vi "Start Animation.vi"(8 "Error In":errorcluster, 11 "Animation Config":T1) -> (0 "Error Out":errorcluster, 3 "Animation Config":T1)   [LabVIEW 2011, in "LMH-Toolbox.lvlib" / "LMH GUI Tools.lvlib"]
uses:
  LMH GUI Tools.lvlib
  Private/Animations/Type Defs/Animation Config.ctl
  <vilib>/picture/picture.llb/imagedata.ctl
  Private/Animations/FGVs/Type Defs/Animation FGV State.ctl
  LMH-Toolbox.lvlib
panel:
  in  "Error In 2":errorcluster
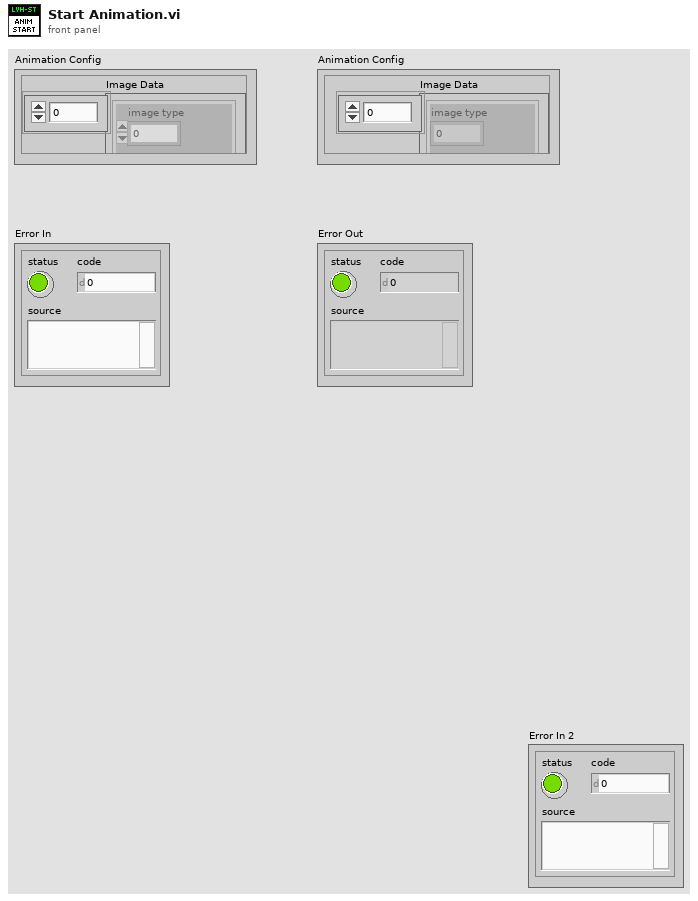
[diagram p1: front panel]
types:
  T1 = typedef "LMH-Toolbox.lvlib/LMH GUI Tools.lvlib/Animation Config.ctl" = cluster{"Image Data":T2[], "Animation Picture Indicator":refnum<vi>, "FPS":u32, "Position":cluster{"X":i16, "Y":i16}}
  T2 = typedef "imagedata.ctl" = cluster{"image type":i32, "image depth":i32, "image":u8[], "mask":u8[], "colors":u32[], "Rectangle":cluster{"left":i16, "top":i16, "right":i16, "bottom":i16}}
  T3 = enum32{"invalid app kind", "Development System", "Run Time System", "Student Edition", "Embedded LabVIEW", "Evaluation", "Custom"}
  T4 = typedef "LMH-Toolbox.lvlib/LMH GUI Tools.lvlib/Animation FGV State.ctl" = enum16{"Init", "Set", "Get"}
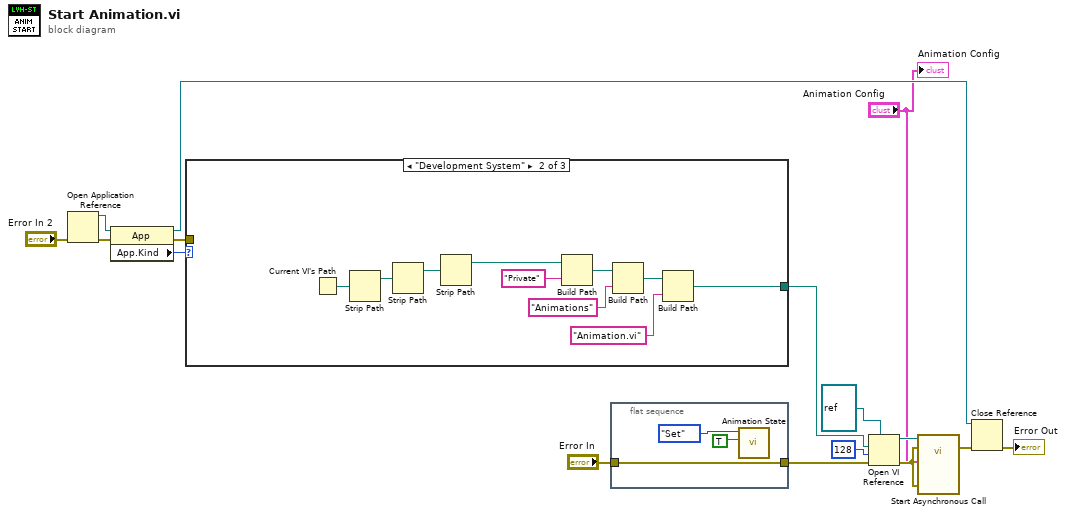
[diagram p0: block diagram]
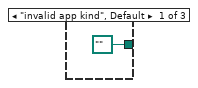
[diagram p2: hidden frame]
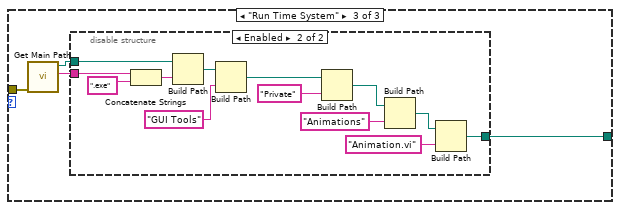
[diagram p3: hidden frame]
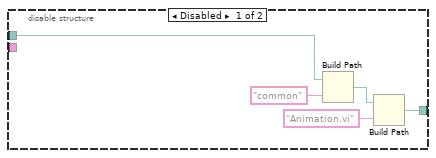
[diagram p4: hidden frame]
diagram:
  n1 = Open Application Reference(8:"Error In 2") -> (0:w11:errorcluster, 3:w10:refnum<vi>)  [unwired: 3 in]
  n2 = property class="App"(reference=w10, error in=w11) -> (reference out=w5:refnum<vi>, error out=w7:errorcluster, "App.Kind"=w9:T3)
  n3 = case shown="\"Development System\"" w9 {
    tunnel: [path "" ("appended path") w22 w29] -> w8
    tunnel: w7 -> [_ _ w30]
    frame "invalid app kind", Default {
    }
    frame "Development System" {
      n4 = Current VI's Path() -> (path=w27:path)
      n5 = Strip Path(path=w27) -> (stripped path=w24:path)  [unwired: 1 out]
      n6 = Strip Path(path=w24) -> (stripped path=w25:path)  [unwired: 1 out]
      n7 = Strip Path(path=w25) -> (stripped path=w19:path)  [unwired: 1 out]
      n8 = Build Path(base path=w19, name or relative path="Private") -> (appended path=w18:path)
      n9 = Build Path(base path=w18, name or relative path="Animations") -> (appended path=w26:path)
      n10 = Build Path(base path=w26, name or relative path="Animation.vi") -> (appended path=w22:path)
    }
    frame "Run Time System" {
      n11 = call "Get Main Path.vi"("Error In"=w30) -> ("Main Name"=w28:string, "Main Dir"=w31:path)  [unwired: 8 in, 1 out]
      n12 = disable-structure shown="Enabled" {
        disable-tunnel: w31 -> [w36 w41]
        disable-tunnel: [w32 w45] -> w29
        disable-tunnel: w28 -> [_ w39]
        frame Disabled {
          n13 = Build Path(base path=w36, name or relative path="common") -> (appended path=w33:path)
          n14 = Build Path(base path=w33, name or relative path="Animation.vi") -> (appended path=w32:path)
        }
        frame Enabled {
          n15 = Concatenate Strings(w39, ".exe" ("string")) -> (w38:string)
          n16 = Build Path(base path=w41, name or relative path=w38) -> (appended path=w42:path)
          n17 = Build Path(base path=w42, name or relative path="GUI Tools") -> (appended path=w44:path)
          n18 = Build Path(base path=w44, name or relative path="Private") -> (appended path=w37:path)
          n19 = Build Path(base path=w37, name or relative path="Animations") -> (appended path=w43:path)
          n20 = Build Path(base path=w43, name or relative path="Animation.vi") -> (appended path=w45:path)
        }
      }
    }
  }
  n21 = flat-sequence {
    tunnel: [w50] -> w14
    tunnel: "Error In" -> [w50]
    frame #0 {
      n22 = call "Animation State.vi"("Running?"=TRUE, "Function"=Animation_FGV_State."Set") -> ()  [unwired: 9 in, 1 out]
    }
  }
  n23 = Open VI Reference(type specifier VI Refnum (for type only)=refnum<vi> refnum, vi path=w8, options=128, error in (no error)=w14) -> (vi reference=w4:refnum<vi>, error out=w3:errorcluster)  [unwired: 2 in]
  n24 = call-by-ref "Start Asynchronous Call"(reference=w4, error in=w3, "Error In"=w3, "Animation Config"="Animation Config") -> (error out=w2:errorcluster)  [unwired: 8 in, 3 out]
  n25 = Close Reference(reference=w5, error in (no error)=w2) -> (error out=→"Error Out":errorcluster)
  "Animation Config" <- "Animation Config"
